vi "Time to Close Switch (SubVI).vi"(4 "data":bool, 5 "Current Limit":dbl=0.2 format="%#_13g", 7 "Voltage Limit":dbl=24.0 format="%#_13g", 8 "Output On (T)":bool=TRUE, 9 "VISA":refnum<visa-resource-name>="COM6", 10 "GEN Addr":i16=6, 11 "BAUD":u16(ring)=4 items=["1200", "2400", "4800", "9600", "19200"]) -> (1 "x-y":dbl)   [LabVIEW 2014]
uses:
  <instrlib>/niDMM/nidmm.llb/niDMM Function.ctl
  <instrlib>/niDMM/nidmm.llb/niDMM Resolution in Digits.ctl
  <vilib>/Utility/error.llb/DialogType.ctl
  <vilib>/DAQmx/create/channels.llb/DAQmx Create Channel (DO-Digital Output).vi
  <vilib>/DAQmx/write.llb/DAQmx Write (Digital Bool 1Line 1Point).vi
  <instrlib>/niDMM/nidmm.llb/niDMM Configure Measurement Digits.vi
panel:
  in  "error":errorcluster
  out "error out":errorcluster
  out "Measurement":dbl format="%.5f"
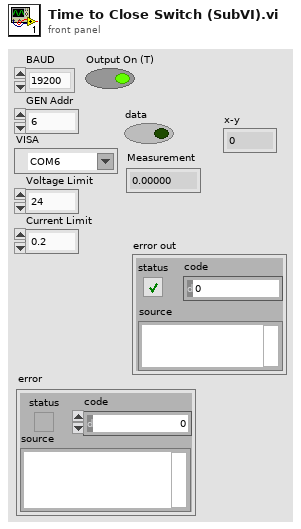
[diagram p1: front panel]
types:
  T1 = typedef "niDMM Function.ctl" = enum16{"DC Volts", "AC Volts", "DC Current", "AC Current", "2-wire Resistance", "4-wire Resistance", "Diode", "Frequency", "Period", "AC Volts DC Coupled", "Capacitance", "Inductance", "Temperature"}
  T2 = typedef "niDMM Resolution in Digits.ctl" = dbl
  T3 = typedef "DialogType.ctl" = u16
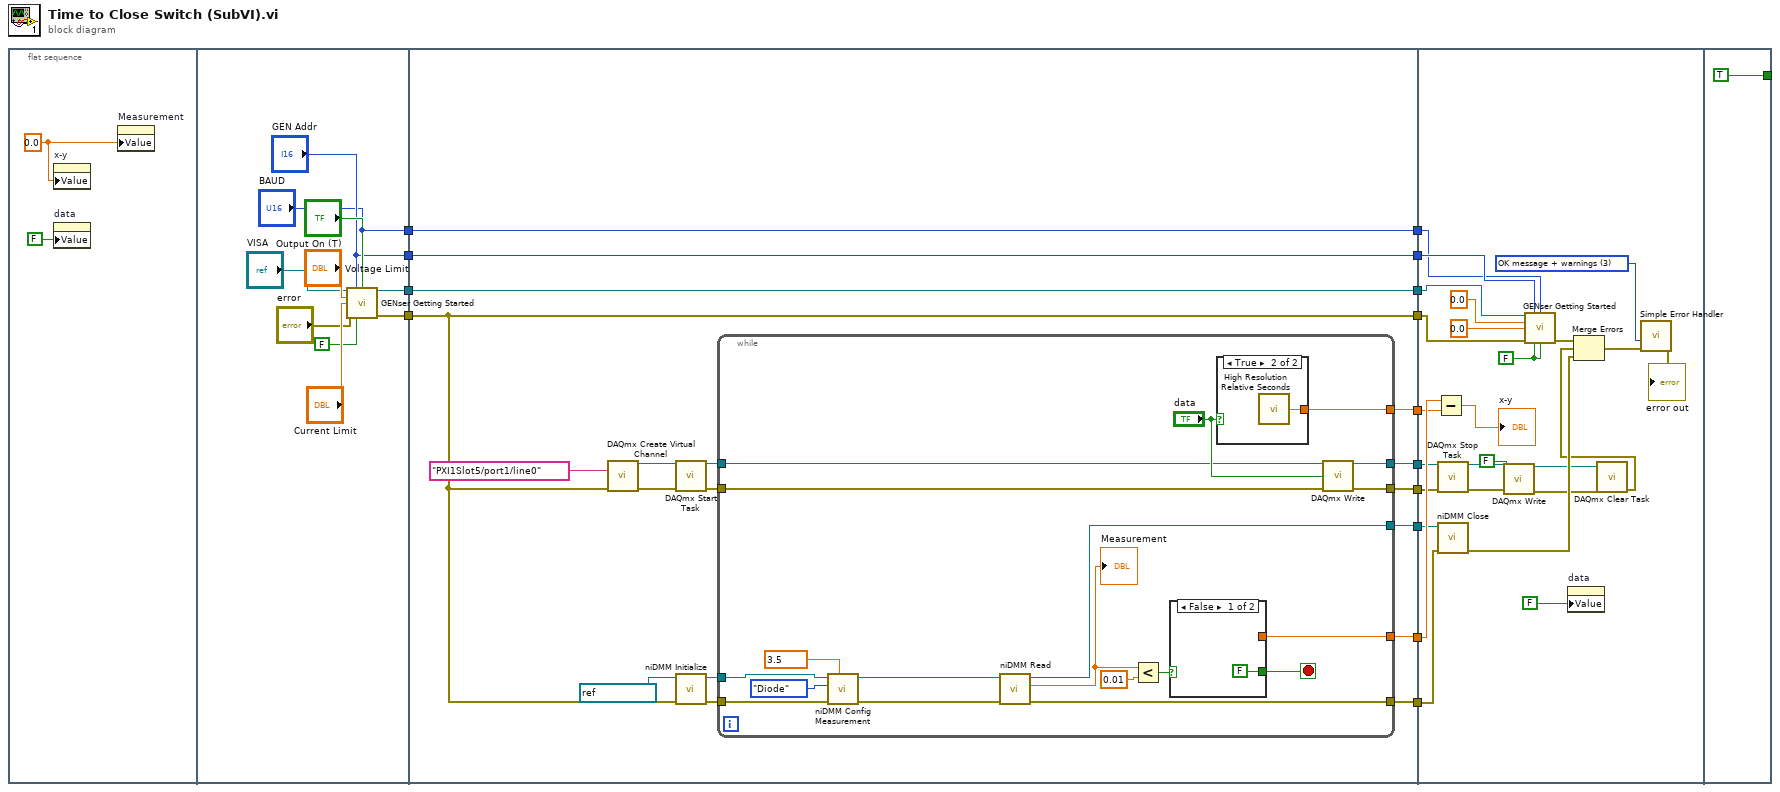
[diagram p0: block diagram]
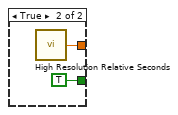
[diagram p2: hidden frame]
diagram:
  n1 = flat-sequence {
    tunnel: [w21] -> w14
    tunnel: ["GEN Addr"] -> w13
    tunnel: ["BAUD"] -> w12
    tunnel: [w18] -> w11
    tunnel: [w44] -> w10
    tunnel: [w43] -> w9
    tunnel: [w42] -> w8
    tunnel: [w41] -> w7
    tunnel: [w40] -> w6
    tunnel: [w28] -> w5
    tunnel: [w39] -> w4
    tunnel: w14 -> [w39]
    tunnel: w13 -> [w38]
    tunnel: [w38] -> w3
    tunnel: [w37] -> w2
    tunnel: w12 -> [w37]
    tunnel: w11 -> [w27]
    tunnel: [w27] -> w1
    tunnel: w10 -> [w90]
    tunnel: w9 -> [w91]
    tunnel: w8 -> [w86]
    tunnel: w7 -> [w88]
    tunnel: w6 -> [w87]
    tunnel: w5 -> [w85]
    tunnel: w4 -> [w82]
    tunnel: w3 -> [w81]
    tunnel: w2 -> [w80]
    tunnel: w1 -> [w77]
    tunnel: [TRUE] -> _
    frame #0 {
      w15 = 0.0 ("x-y")
      n2 = property on="x-y" class="DigNum (strict)"("Value"=w15) -> ()  [unwired: 2 in, 2 out]
      n3 = property on="data" class="Bool (strict)"("Value"=FALSE ("data")) -> ()  [unwired: 2 in, 2 out]
      n4 = property on="Measurement" class="DigNum (strict)"("Value"=w15) -> ()  [unwired: 2 in, 2 out]
    }
    frame #1 {
      n5 = call "GENser Getting Started.vi"("VISA"="VISA", "GEN Addr"="GEN Addr", "BAUD"="BAUD", "Voltage Limit"="Voltage Limit", "Current Limit"="Current Limit", "error"="error", "Reset (T)"=FALSE, "Output On (T)"="Output On (T)") -> ("VISA out"=w21:refnum<visa-resource-name>, "error out"=w18:errorcluster)  [unwired: 4 in, 2 out]
    }
    frame #2 {
      n6 = call-poly <vilib>:"DAQmx Create Virtual Channel.vi"("lines"=tag "PXI1Slot5/port1/line0", "error in"=w27) -> ("task out"=w32:refnum<k21>, "error out"=w33:errorcluster)  [unwired: 12 in]
      n7 = call <vilib>:"DAQmx Start Task.vi"("task/channels in"=w32, "error in"=w33) -> ("task out"=w30:refnum<k21>, "error out"=w29:errorcluster)  [unwired: 12 in]
      n8 = call <instrlib>:"niDMM Initialize.vi"("error in (no error)"=w27, "Instrument Descriptor"=refnum<k15> "PXI1Slot9") -> ("error out"=w34:errorcluster, "instrument handle out"=w35:refnum<k15>)  [unwired: 8 in]
      n9 = while {
        tunnel: [w60] -> w44
        tunnel: [w59] -> w43
        tunnel: [w46] -> w42
        tunnel: [w57] -> w41
        tunnel: [w56] -> w40
        tunnel: [w45] -> w28
        tunnel: w35 -> [w50]
        tunnel: w34 -> [w49]
        tunnel: w30 -> [w55]
        tunnel: w29 -> [w54]
        stop <- w58 stop-if-true
        w63 = T2 3.5 items=["3 1/2"=3.5, "4 1/2"=4.5, "5 1/2"=5.5, "6 1/2"=6.5, "7 1/2"=7.5] ("Resolution in Digits")
        n10 = call-poly <instrlib>:"niDMM Config Measurement.vi"("Resolution in Digits"=w63, "error in (no error)"=w49, "Function"=niDMM_Function."Diode", "instrument handle"=w50) -> ("error out"=w47:errorcluster, "instrument handle out"=w48:refnum<k15>)  [unwired: 6 in]
        n11 = call <instrlib>:"niDMM Read.vi"("error in (no error)"=w47, "instrument handle"=w48) -> ("error out"=w45:errorcluster, "Measurement"=w52:dbl, "instrument handle out"=w46:refnum<k15>)  [unwired: 7 in]
        "Measurement" <- w52
        n12 = Less?(x=w52, y=0.01) -> (x < y?=w53:bool)
        n13 = case shown="False" w53 {
          tunnel: [_ w66] -> w59
          tunnel: [FALSE TRUE] -> w58
          frame False {
          }
          frame True {
            n14 = call <vilib>:"High Resolution Relative Seconds.vi"() -> ("relative seconds"=w66:dbl)
          }
        }
        n15 = case shown="True" "data" {
          tunnel: [_ w67] -> w60
          frame False {
          }
          frame True {
            n16 = call <vilib>:"High Resolution Relative Seconds.vi"() -> ("relative seconds"=w67:dbl)
          }
        }
        n17 = call-poly <vilib>:"DAQmx Write.vi"("task/channels in"=w55, "data"="data", "error in"=w54) -> ("task out"=w57:refnum<k21>, "error out"=w56:errorcluster)  [unwired: 10 in, 1 out]
      }
    }
    frame #3 {
      w75 = FALSE ("Reset (T)")
      w92 = T3 3 items=["no dialog", "OK message", "continue or stop message", "OK message + warnings", "continue/stop + warnings"] ("type of dialog (OK msg:1)")
      n18 = Subtract(x=w91, y=w90) -> (x-y=→"x-y":dbl)
      n19 = call <vilib>:"DAQmx Stop Task.vi"("task/channels in"=w88, "error in"=w87) -> ("task out"=w73:refnum<k21>, "error out"=w72:errorcluster)  [unwired: 12 in]
      n20 = call <instrlib>:"niDMM Close.vi"("error in (no error)"=w85, "instrument handle"=w86) -> ("error out"=w83:errorcluster)  [unwired: 9 in]
      n21 = call-poly <vilib>:"DAQmx Write.vi"("task/channels in"=w73, "data"=FALSE, "error in"=w72) -> ("task out"=w70:refnum<k21>, "error out"=w71:errorcluster)  [unwired: 10 in, 1 out]
      n22 = call "GENser Getting Started.vi"("VISA"=w82, "GEN Addr"=w81, "BAUD"=w80, "Voltage Limit"=0.0, "Current Limit"=0.0, "error"=w77, "Reset (T)"=w75, "Output On (T)"=w75) -> ("error out"=w76:errorcluster)  [unwired: 4 in, 3 out]
      n23 = property on="data" class="Bool (strict)"("Value"=FALSE ("data")) -> ()  [unwired: 2 in, 2 out]
      n24 = call <vilib>:"DAQmx Clear Task.vi"("task in"=w70, "error in"=w71) -> ("error out"=w69:errorcluster)  [unwired: 13 in]
      n25 = Merge Errors(w76, w69, w83) -> (w84:errorcluster)
      "error out" <- w84
      n26 = call <vilib>:"Simple Error Handler.vi"("type of dialog (OK msg:1)"=w92, "error in (no error)"=w84) -> ()  [unwired: 3 in, 5 out]
    }
    frame #4 {
    }
  }
